vi "Koheras_Laser_ON-OFF-switch.vi"(8 "error in":errorcluster, 10 "Koheras Seed Laser":bool, 11 "VISA resource name in":refnum<visa-resource-name>) -> (0 "error out":errorcluster, 2 "Return":string[](array[string]), 3 "VISA resource name out":refnum<visa-resource-name>)   [LabVIEW 2011]
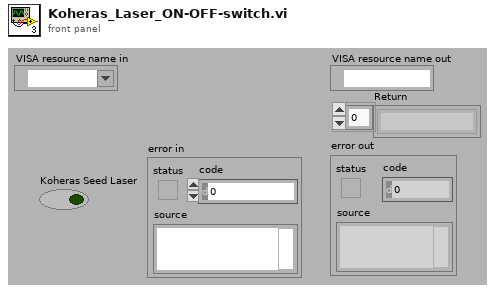
[diagram p1: front panel]
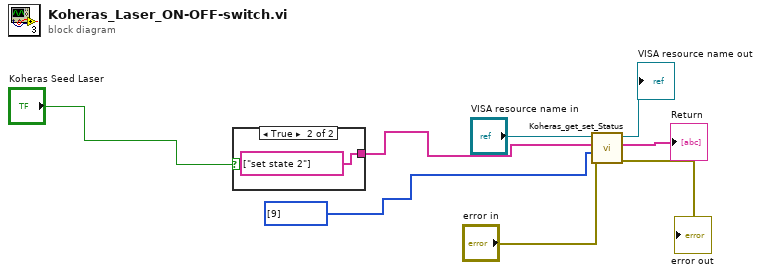
[diagram p0: block diagram]
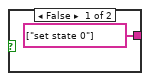
[diagram p2: hidden frame]
diagram:
  n1 = case shown="True" "Koheras Seed Laser" {
    tunnel: [string[] ["set state 0"] string[] ["set state 2"]] -> w6
    frame False {
    }
    frame True {
    }
  }
  n2 = call "Koheras_get_set_Status.vi"("error in"="error in", "Array 2"=i32[] [9], "Array"=w6, "VISA resource name in"="VISA resource name in") -> ("error out"=→"error out":errorcluster, "Return"=→"Return":string[], "VISA resource name out"=→"VISA resource name out":refnum<visa-resource-name>)  [unwired: 5 in]
